vi "UTF-8 To Encoded String.vi"(8 "error in (no error)":errorcluster, 10 "UTF-8 string":string, 11 "Encoding in":refnum<class "CConfig Automatic Encoding.lvclass">) -> (0 "error out":errorcluster, 2 "Encoded string":string, 3 "Encoding out":refnum<class "CConfig Automatic Encoding.lvclass">)   [LabVIEW 2013, in "CConfig Automatic Encoding.lvclass"]
doc: "Copyright 2018, Carya Automatisering, Wiebe Walstra."
uses:
  CConfig Automatic Encoding.lvclass
  CConfig Automatic Encoding.lvclass/CConfig Automatic Encoding.ctl
  CConfig Encoding.lvclass
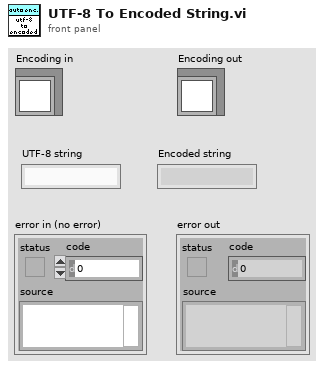
[diagram p1: front panel]
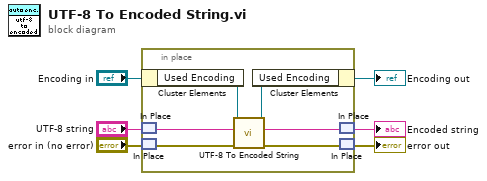
[diagram p0: block diagram]
diagram:
  n1 = in-place {
    n2 = in-place-cluster #1("Encoding in") -> ("Used Encoding"=w12:refnum<class "CConfig Encoding.lvclass">)
    n3 = in-place-match #2("UTF-8 string") -> (w10:string)
    n4 = in-place-match #3("error in (no error)") -> (w8:errorcluster)
    n5 = call-dynamic "UTF-8 To Encoded String.vi"("error in (no error)"=w8, "UTF-8 string"=w10, "Encoding in"=w12) -> ("error out"=w7:errorcluster, "Encoded string"=w9:string, "Encoding out"=w11:refnum<class "CConfig Encoding.lvclass">)  [unwired: 6 in]
    n6 = in-place-cluster #1("Used Encoding"=w11) -> (→"Encoding out":refnum<class "CConfig Automatic Encoding.lvclass">)
    n7 = in-place-match #2(w9) -> (→"Encoded string":string)
    n8 = in-place-match #3(w7) -> (→"error out":errorcluster)
  }
